vi "Enter Remote Mode.vi"(8 "error in (no error)":errorcluster, 11 "ASIA Pump #":i32) -> (0 "error out":errorcluster, 2 "Completed":bool=TRUE, 3 "ASIA Pump #":i32)   [LabVIEW 2018, in "ASIA Pump.lvlib"]
uses:
  ASIA Pump.lvlib
  Program Files (x86)/Pfizer/FAST/data/AsiaPumpInterface.dll
panel:
  out "error out 2":errorcluster
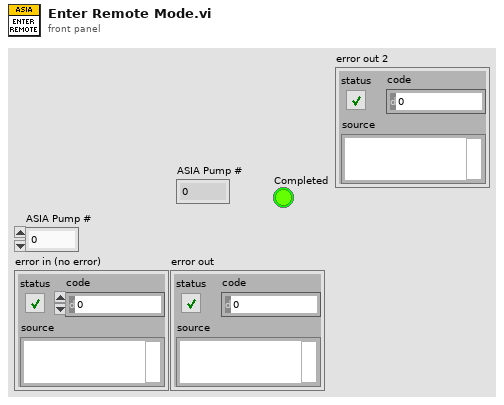
[diagram p1: front panel]
types:
  T1 = cluster{"Busy":bool, "PumpCnt":dbl, "RemoteEntered":bool, "OverpressureSet":bool}[]
  T2 = cluster{"Busy":bool, "PumpCnt":dbl, "RemoteEntered":bool, "OverpressureSet":bool}
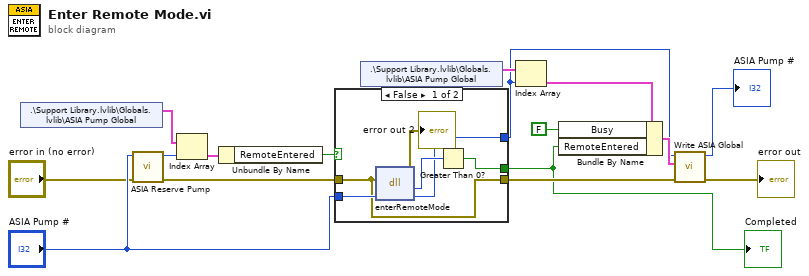
[diagram p0: block diagram]
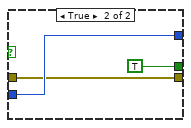
[diagram p2: hidden frame]
diagram:
  n1 = shared-variable ".\\Support Library.lvlib\\Globals.lvlib\\ASIA Pump Global"() -> (w16:T1)  [unwired: 1 in, 1 out]
  n2 = call "ASIA Reserve Pump.vi"("error in (no error)"="error in (no error)", "ASIA Pump #"="ASIA Pump #") -> ("error out"=w10:errorcluster, "ASIA Pump #"=w12:i32)  [unwired: 8 in]
  n3 = Index Array(array=w16, index=w12) -> (element=w15:T2)
  n4 = Unbundle By Name(w15) -> ("RemoteEntered"=w14:bool)
  n5 = case shown="False" w14 {
    tunnel: w10 -> [w18 w23]
    tunnel: "ASIA Pump #" -> [w22 w24]
    tunnel: [w20 TRUE] -> w3
    tunnel: [w19 w24] -> w5
    tunnel: [w18 w23] -> w6
    frame False {
      n6 = dll-call lib="C:/Program Files (x86)/Pfizer/FAST/data/AsiaPumpInterface.dll" fn="enterRemoteMode"(error in=w18, "pumpNum"=w22) -> (error out=→"error out 2":errorcluster, "return type"=w21:i8, "pumpNum"=w19:u32)  [unwired: 2 in, 1 out]
      n7 = Greater Than 0?(x=w21) -> (x > 0?=w20:bool)
    }
    frame True {
    }
  }
  "Completed" <- w3
  n8 = shared-variable ".\\Support Library.lvlib\\Globals.lvlib\\ASIA Pump Global"() -> (w8:T1)  [unwired: 1 in, 1 out]
  n9 = Index Array(array=w8, index=w5) -> (element=w9:T2)
  n10 = Bundle By Name(cluster=w9, "Busy"=FALSE, "RemoteEntered"=w3) -> (w7:T2)
  n11 = call "Write ASIA Global.vi"("error in (no error)"=w6, "ASIA Global"=w7, "Pump Number"=w5) -> ("error out"=→"error out":errorcluster, "Pump Number"=→"ASIA Pump #":i32)  [unwired: 7 in]
